vi "MS5607_Main.vi"(8 "Error In":errorcluster, 11 "Enum":T1) -> (0 "error out":errorcluster, 2 "MS5607_TempC 3":dbl format="%#.2g", 3 "MS5607_Pressure_mbar 3":dbl format="%#.2f")   [LabVIEW 2016]
uses:
  MS5607_StateMachine.ctl
  <vilib>/myRIO/Instrument Drivers/Onboard IO/I2C/vis/Configure.vi
  <vilib>/myRIO/Instrument Drivers/Onboard IO/I2C/vis/Write.vi
  <vilib>/myRIO/Instrument Drivers/Onboard IO/I2C/vis/Smart Open.vi
  <vilib>/Utility/error.llb/Error Cluster From Error Code.vi
  <vilib>/myRIO/Common/Instrument Driver Framework/myRIO v1.0/I2C/vis/myRIO v1.0 Configure I2C.vi
  <vilib>/myRIO/Common/Instrument Driver Framework/myRIO v1.0/I2C/vis/myRIO v1.0 Write I2C.vi
panel:
  out "dT 2":dbl
  out "SENS 2":dbl
  out "OFF 2":dbl
  out "Calibration Values":T2
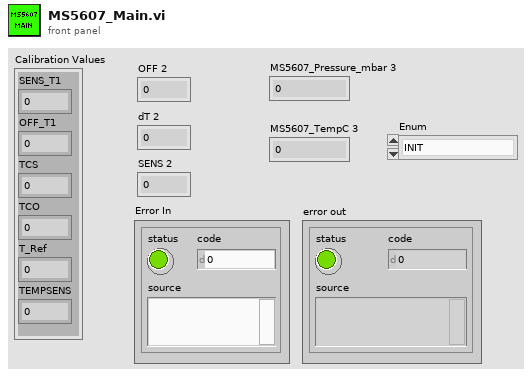
[diagram p1: front panel]
types:
  T1 = typedef "MS5607_StateMachine.ctl" = enum16{"INIT", "GET_CALI_BYTE", "GET_SENSOR_DATA", "CALC_RAW_DATA", "END", "ERROR"}
  T2 = cluster{"SENS_T1":u16, "OFF_T1":u16, "TCS":u16, "TCO":u16, "T_Ref":u16, "TEMPSENS":u16}
  T3 = cluster{"Raw Pressure Data":u32, "Raw Temperature Data":u32}
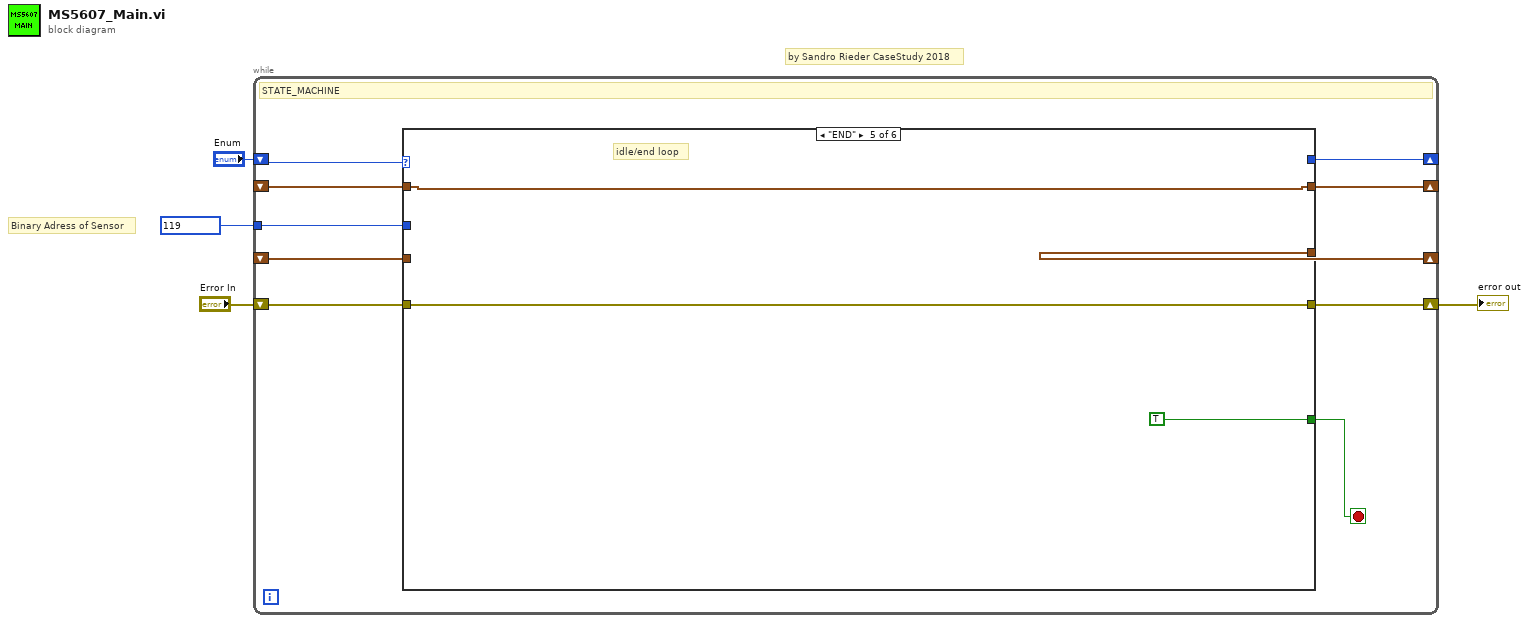
[diagram p0: block diagram]
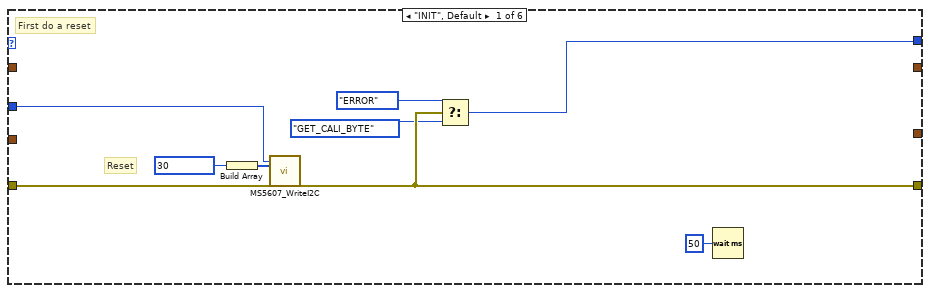
[diagram p2: hidden frame]
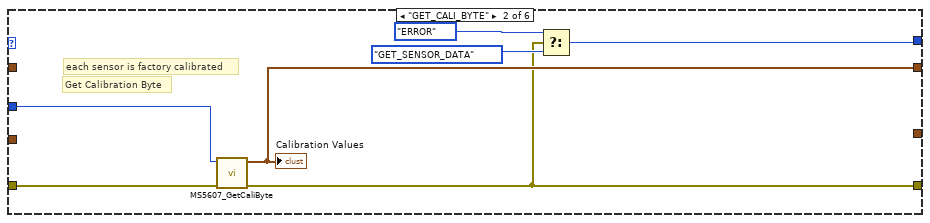
[diagram p3: hidden frame]
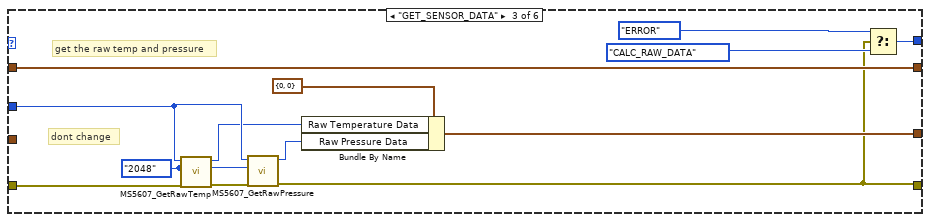
[diagram p4: hidden frame]
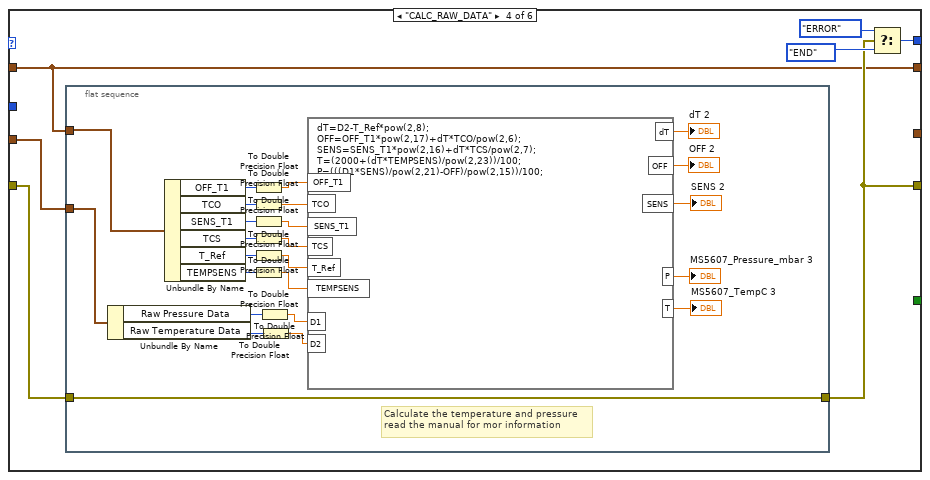
[diagram p5: hidden frame]
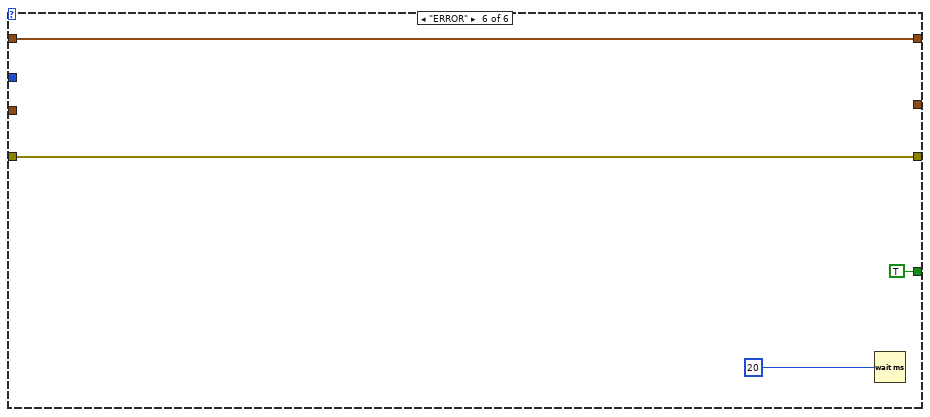
[diagram p6: hidden frame]
diagram:
  # "Binary Adress of Sensor"
  # "by Sandro Rieder CaseStudy 2018"
  n1 = while {
    shift-right: [w6] -> w3
    shift-left: "Error In" -> [w13]
    shift-right: [w12] -> _
    shift-left: "Enum" -> [w14]
    shift-right: [w11] -> _
    shift-left: _ -> [w10]
    tunnel: u8 119 -> [w9]
    shift-right: [w8] -> _
    shift-left: _ -> [w7]
    stop <- w5 stop-if-true
    # "STATE_MACHINE"
    n2 = case shown="\"END\"" w14 {
      tunnel: w13 -> [w21 w30 w43 w46 w77 w81]
      tunnel: [w20 w26 w31 w45 w77 w81] -> w6
      tunnel: [w17 w28 w33 w47 _ _] -> w12
      tunnel: [_ w29 w32 w44 w76 w79] -> w11
      tunnel: w10 -> [_ _ w32 w44 w76 w79]
      tunnel: w9 -> [w16 w24 w40 _ _ _]
      tunnel: [_ _ w36 _ _ _] -> w8
      tunnel: w7 -> [_ _ _ w50 _ _]
      tunnel: [_ _ _ _ TRUE TRUE] -> w5
      frame "INIT", Default {
        # "First do a reset"
        # "Reset"
        n3 = Build Array(u8 30) -> (w23:u8[])
        n4 = call "MS5607_WriteI2C.vi"("Slave Address (7-bit)"=w16, "Bytes to Write"=w23, "error in (no error)"=w21) -> ("error out"=w20:errorcluster)  [unwired: 24 in]
        n5 = Select(t=MS5607_StateMachine."ERROR", s=w20, f=MS5607_StateMachine."GET_CALI_BYTE") -> (s? t:f=w17:T1)
        n6 = Wait (ms)(milliseconds to wait=u32 50) -> ()  [unwired: 1 out]
      }
      frame "GET_CALI_BYTE" {
        # "each sensor is factory calibrated"
        # "Get Calibration Byte"
        n7 = call "MS5607_GetCaliByte.vi"("error in (no error)"=w30, "Numeric"=w24) -> ("error out"=w26:errorcluster, "Calibration Values"=w29:T2)  [unwired: 8 in]
        "Calibration Values" <- w29
        n8 = Select(t=MS5607_StateMachine."ERROR", s=w26, f=MS5607_StateMachine."GET_SENSOR_DATA") -> (s? t:f=w28:T1)
      }
      frame "GET_SENSOR_DATA" {
        w42 = enum8{"256", "512", "1024", "2048"}."2048" ("OSR")
        # "get the raw temp and pressure"
        # "dont change"
        n9 = call "MS5607_GetRawTemp.vi"("error in (no error)"=w43, "OSR"=w42, "Slave Address (7-bit)"=w40) -> ("error out"=w41:errorcluster, "Raw Temperature Data"=w37:u32)  [unwired: 7 in]
        n10 = call "MS5607_GetRawPressure.vi"("error in (no error)"=w41, "OSR"=w42, "Slave Address (7-bit)"=w40) -> ("error out"=w31:errorcluster, "Raw Pressure Data"=w38:u32)  [unwired: 7 in]
        n11 = Bundle By Name(cluster=T3 {"Raw Pressure Data"=0, "Raw Temperature Data"=0}, "Raw Temperature Data"=w37, "Raw Pressure Data"=w38) -> (w36:T3)
        n12 = Select(t=MS5607_StateMachine."ERROR", s=w31, f=MS5607_StateMachine."CALC_RAW_DATA") -> (s? t:f=w33:T1)
      }
      frame "CALC_RAW_DATA" {
        n13 = flat-sequence {
          tunnel: w50 -> [w55]
          tunnel: w44 -> [w52]
          tunnel: w46 -> [w51]
          tunnel: [w51] -> w45
          frame #0 {
            # "Calculate the temperature and pressure\nread the manual for mor information"
            n14 = Unbundle By Name(w55) -> ("Raw Pressure Data"=w54:u32, "Raw Temperature Data"=w53:u32)
            n15 = Unbundle By Name(w52) -> ("OFF_T1"=w74:u16, "TCO"=w73:u16, "SENS_T1"=w72:u16, "TCS"=w71:u16, "T_Ref"=w62:u16, "TEMPSENS"=w61:u16)
            n16 = To Double Precision Float(number=w74) -> (double precision float=w69:dbl)
            n17 = To Double Precision Float(number=w73) -> (double precision float=w68:dbl)
            n18 = To Double Precision Float(number=w72) -> (double precision float=w67:dbl)
            n19 = To Double Precision Float(number=w71) -> (double precision float=w66:dbl)
            n20 = To Double Precision Float(number=w62) -> (double precision float=w60:dbl)
            n21 = To Double Precision Float(number=w61) -> (double precision float=w59:dbl)
            n22 = To Double Precision Float(number=w54) -> (double precision float=w70:dbl)
            n23 = To Double Precision Float(number=w53) -> (double precision float=w56:dbl)
            n24 = formula code="dT=D2-T_Ref*pow(2,8);\nOFF=OFF_T1*pow(2,17)+dT*TCO/pow(2,6);      \nSENS=SENS_T1*pow(2,16)+dT*TCS/pow(2,7);\nT=(2000+(dT*TEMPSENS)/pow(2,23))/100;   \nP=(((D1*SENS)/pow(2,21)-OFF)/pow(2,15))/100;"("OFF_T1"=w69, "TCO"=w68, "SENS_T1"=w67, "TCS"=w66, "D1"=w70, "T_Ref"=w60, "TEMPSENS"=w59, "D2"=w56) -> ("OFF"=→"OFF 2":dbl, "SENS"=→"SENS 2":dbl, "P"=→"MS5607_Pressure_mbar 3":dbl, "T"=→"MS5607_TempC 3":dbl, "dT"=→"dT 2":dbl)
          }
        }
        n25 = Select(t=MS5607_StateMachine."ERROR", s=w45, f=MS5607_StateMachine."END") -> (s? t:f=w47:T1)
      }
      frame "END" {
        # "idle/end loop"
      }
      frame "ERROR" {
        n26 = Wait (ms)(milliseconds to wait=u32 20) -> ()  [unwired: 1 out]
      }
    }
  }
  "error out" <- w3
